vi "Periodic Tasks.vi"(8 "error in":errorcluster) -> ()   [LabVIEW 2015]
doc: "This VI runs in parallel to other tasks. It can contain as many user-defined periodic loops as you need. These can carry out PID or other sorts of timed response."
uses:
  Common Code/Goal Vision Packet.ctl
  Common Code/Change Detect Int.vi
  Common Code/Utilities/TimeManager.vi
  Common Code/Change Detect Boolean.vi
  Robot Global Data.vi
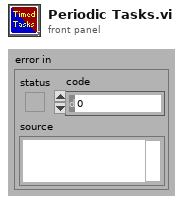
[diagram p1: front panel]
types:
  T1 = typedef "WPI_MotorControlDeviceRef.ctl" = cluster{"DeviceStatus":errorcluster, "Type":T2, "PWM":cluster{"PWM Channel":T3, "DeadBand":T4}, "CAN":cluster{"Device Number":u8, "Control Mode":T5, "Semaphore":T6, "Max Vout":dbl, "TalonSRX Control Mode":T7}, "Invert":bool}
  T2 = typedef "WPI_MotorControlType.ctl" = enum16{"PWM", "CAN", "CANTalonSRX"}
  T3 = typedef "FPGA_DIOPWMChannel.ctl" = enum8{"PWM 0", "PWM 1", "PWM 2", "PWM 3", "PWM 4", "PWM 5", "PWM 6", "PWM 7", "PWM 8", "PWM 9", "PWM MXP 0", "PWM MXP 1", "PWM MXP 2", "PWM MXP 3", "PWM MXP 4", "PWM MXP 5", "PWM MXP 6", "PWM MXP 7", "PWM MXP 8", "PWM MXP 9", "Invalid"}
  T4 = typedef "WPI_PWMDeadband.ctl" = cluster{"Name":string, "maxPositivePwm":i32, "minPositivePwm":i32, "centerPwm":i32, "maxNegativePwm":i32, "minNegativePwm":i32, "angularRange":u16}
  T5 = typedef "WPI_CANJaguar_ControlMode.ctl" = enum8{"Percent VBus", "Current", "Speed", "Position", "Voltage"}
  T6 = typedef "Semaphore RefNum" = refnum<k1>
  T7 = typedef "WPI_CANTalonSRX_APIControlMode.ctl" = enum8{"Percent VBus", "Speed", "Position", "Slave", "Unchanged / Invalid", "Voltage Compensation", "Current", "Motion Profile"}
  T8 = typedef "WPI_DriverStationRobotMode2.ctl" = enum16{"Autonomous Disabled", "Autonomous Enabled", "Teleop Disabled", "Teleop Enabled", "Disconnected", "Finish", "Test Disabled", "Test Enabled", "Emergency Stopped"}
  T9 = typedef "Shooter State Cluster.ctl" = cluster{"State":T10, "Left RPM":dbl, "Right RPM":dbl, "Shooter Ready?":bool, "Ball Loaded?":bool, "Current Angle":dbl, "Angle Motor Output":dbl, "Trigger Output":dbl, "Angle Ready?":bool, "RPM Ready?":bool, "Vision Ready?":bool, "Ball Loaded?":bool, "Mode":T11, "Shot Type":T12, "Pot Height":dbl, "Current Tripped Forward?":bool, "Current Tripped Backward?":bool, "Right Servo":i32, "Left Servo":i32, "IR Override":bool, "Intake Danger?":bool, "Intake Angle Ready?":bool}
  T10 = typedef "Shooter State.ctl" = enum16{"Idle", "Settle Ball", "Warmup", "Shooter Ready", "Shoot"}
  T11 = typedef "Shoot Modes Enum.ctl" = enum16{"Manual", "Safe", "Auto"}
  T12 = typedef "Shot Type.ctl" = enum16{"Batter Shot", "Corner Shot", "Cleat Shot", "Vision Shot", "Deep Middle Shot"}
  T13 = typedef "Goal Vision Packet.ctl" = cluster{"Distance":dbl, "Center X":dbl, "Center Y":dbl, "Found Target?":bool, "Robot Center":dbl, "Angle":dbl}
  T14 = typedef "Dashboard Control Data.ctl" = cluster{"Shooter Presets":T15, "Encoder Control":T17, "Steer PID output":cluster{"output high":dbl, "output low":dbl}, " Steer PID gains":cluster{"proportional gain (Kc)":dbl, "integral time (Ti, min)":dbl, "derivative time (Td, min)":dbl}, "Drivetrain Settings":T18, "Vision Packet":T13, "Dashboard Drivetrain Command":T19, "Info/Command Cluster":T21, "Ball Vision Packet":T22, "Intake Presets":T24, "Intake Encoder Control":T26, "Climb Presets":T27, "Goal Output Range":cluster{"output high":dbl, "output low":dbl}, "Enabled Systems":T28, "Auton Presets":T29, "Pressure M":dbl, "Pressure B":dbl, "Vision Timeout":dbl, "Auto-Shift":T30}
  T15 = typedef "Shooter Presets.ctl" = cluster{"Batter Shot":T16, "Deep Middle":T16, "Manual Shot":T16, "Left Ticks Per Rotation":dbl, "Right Ticks Per Rotation":dbl, "Low Bar Shot":T16, "Shooter RPM Tolerance":dbl, "Trigger Power":dbl, "Fire from Load Delay":i32, "Max Angle":dbl, "Min Angle":dbl, "Angle PID gains":cluster{"P":dbl, "I":dbl, "D":dbl}, "Angle Output":cluster{"output high":dbl, "output low":dbl}, "Shooter Angle Tolerance":dbl, "Vision Shoot x^2":dbl, "Vision Shoot x":dbl, "Feed Forward Max Accel":dbl, "Feed Forward Kv":dbl, "Backwards Trigger":dbl, "Shot Finish Delay (ms)":dbl, "Angle Max Current":dbl, "Angle Current Trip Time":dbl, "Intake Angle":dbl, "Vision Shoot c":dbl, "Reset?":bool, "Button Release Delay":dbl, "Angle Pot x":dbl, "Angle Pot c":dbl, "Ignore Angle?":bool, "Max RPM":dbl, "Safty Frist Angle":dbl, "Intake Danger Height":dbl, "Angle Pot B":i32, "Angle Pot M":dbl, "FF Finish RPM":dbl, "RPM PID Right":cluster{"P":dbl, "I":dbl, "D":dbl, "FF":dbl}, "RPM PID Left":cluster{"P":dbl, "I":dbl, "D":dbl, "FF":dbl}, "Backwards RPM":dbl, "Vision RPM":dbl, "Run Wheels Backward Delay":u32, "Cleat Shot":T16, "Vision Far RPM":dbl, "Vision Far Distance":dbl, "Vision Far Angle":dbl}
  T16 = typedef "Shot Presets.ctl" = cluster{"L":dbl, "R":dbl, "A":dbl}
  T17 = typedef "Encoder Control.ctl" = cluster{"Right Tick Constant":dbl, "Left Tick Constant":dbl, "Reset?":bool, "Y Dist":cluster{"PID gains":cluster{"proportional gain (Kc)":dbl, "integral time (Ti, min)":dbl, "derivative time (Td, min)":dbl}}, "Y Stop Thresh":dbl, "Y Stop Speed":dbl}
  T18 = typedef "Drivetrain Settings.ctl" = cluster{"Gyro Tolerance":dbl, "Throttle Ramp (ms)":dbl, "Kv":dbl, "Ka":dbl, "Feed Forward P":dbl, "Feed Forward D":dbl, "Goal Vision PID gains":cluster{"proportional gain (Kc)":dbl, "integral time (Ti, min)":dbl, "derivative time (Td, min)":dbl}, "Goal Detection Window":dbl, "Creep Rate":dbl, "Vision Throttle Threshold":dbl, "Min Turn Output":dbl, "Left Batter Angle":dbl, "Right Batter Angle":dbl}
  T19 = typedef "Dashboard Drivetrain Command.ctl" = cluster{"Drivetrain Vision":T20}
  T20 = typedef "Drivetrain Vision.ctl" = cluster{"Goal Window":dbl, "Ball Window":dbl}
  T21 = typedef "Ball Tracking Command Cluster.ctl" = cluster{"Distance to Ball":dbl, "Desired Angle":dbl, "Command":enum16{"Turn to Ball", "Turn to Angle", "Get Distance"}, "Pixels from Center":dbl}
  T22 = typedef "Ball Vision Packet.ctl" = cluster{"Ball Detected?":bool, "Distance to Ball":dbl, "Desired Angle":dbl, "Pixels from Center":dbl, "Tracking mode":T23}
  T23 = typedef "Tracking Mode.ctl" = enum16{"Turn to Ball", "Turn to Angle"}
  T24 = typedef "Intake Presets.ctl" = cluster{"Intake Speed":dbl, "Outake Speed":dbl, "Low Height":dbl, "Half Height":dbl, "High Idle Height":dbl, "Angle Speed":dbl, "Angle Tolerance":dbl, "Encoder Scale":dbl, "Load Height":dbl, "Output Range":T25, "Rotation Power Max/Min":dbl, "MaxCurrent":dbl, "Intake Trip Time":dbl, "Idle Height":dbl, "Max Height":dbl, "Reset Encoders?":bool, "PID gains":cluster{"proportional gain (Kc)":dbl, "integral time (Ti, min)":dbl, "derivative time (Td, min)":dbl}, "Intake Stop Delay":u32, "Settle Time":dbl, "Settle Wait Time":dbl, "Pull Up Delay":dbl}
  T25 = typedef "Drivetrain Output Range.ctl" = cluster{"output high":dbl, "output low":dbl}
  T26 = typedef "IntakeEcoderControl.ctl" = cluster{"Arm Tick Constant":dbl, "Reset?":bool, "Y Dist":cluster{"PID gains":cluster{"proportional gain (Kc)":dbl, "integral time (Ti, min)":dbl, "derivative time (Td, min)":dbl}}, "Y Stop Thresh":dbl, "Y Stop Speed":dbl}
  T27 = typedef "Climb Presets.ctl" = cluster{"Pull Power":dbl, "Extend Power":dbl}
  T28 = typedef "Enabled Systems.ctl" = cluster{"Shoot":bool, "Intake":bool, "DT":bool, "Gyro":bool, "100ms":bool, "US":bool}
  T29 = typedef "Autonomous Presets.ctl" = cluster{"Pitch Limit":dbl, "Roll Limit":dbl, "Start Position":dbl, "Cross Position":dbl}
  T30 = typedef "Auto Shift Cluster.ctl" = cluster{"Delay":dbl, "Speed Thresh":dbl, "Upshift Accel":dbl, "Upshift Throttle":dbl, "Upshift Throttle Accel":dbl, "Downshift Throttle":dbl, "Downshift Throttle Accel":dbl}
  T31 = typedef "WPI_CameraDevRef.ctl" = cluster{"Camera Address":string, "CameraStatus":errorcluster}
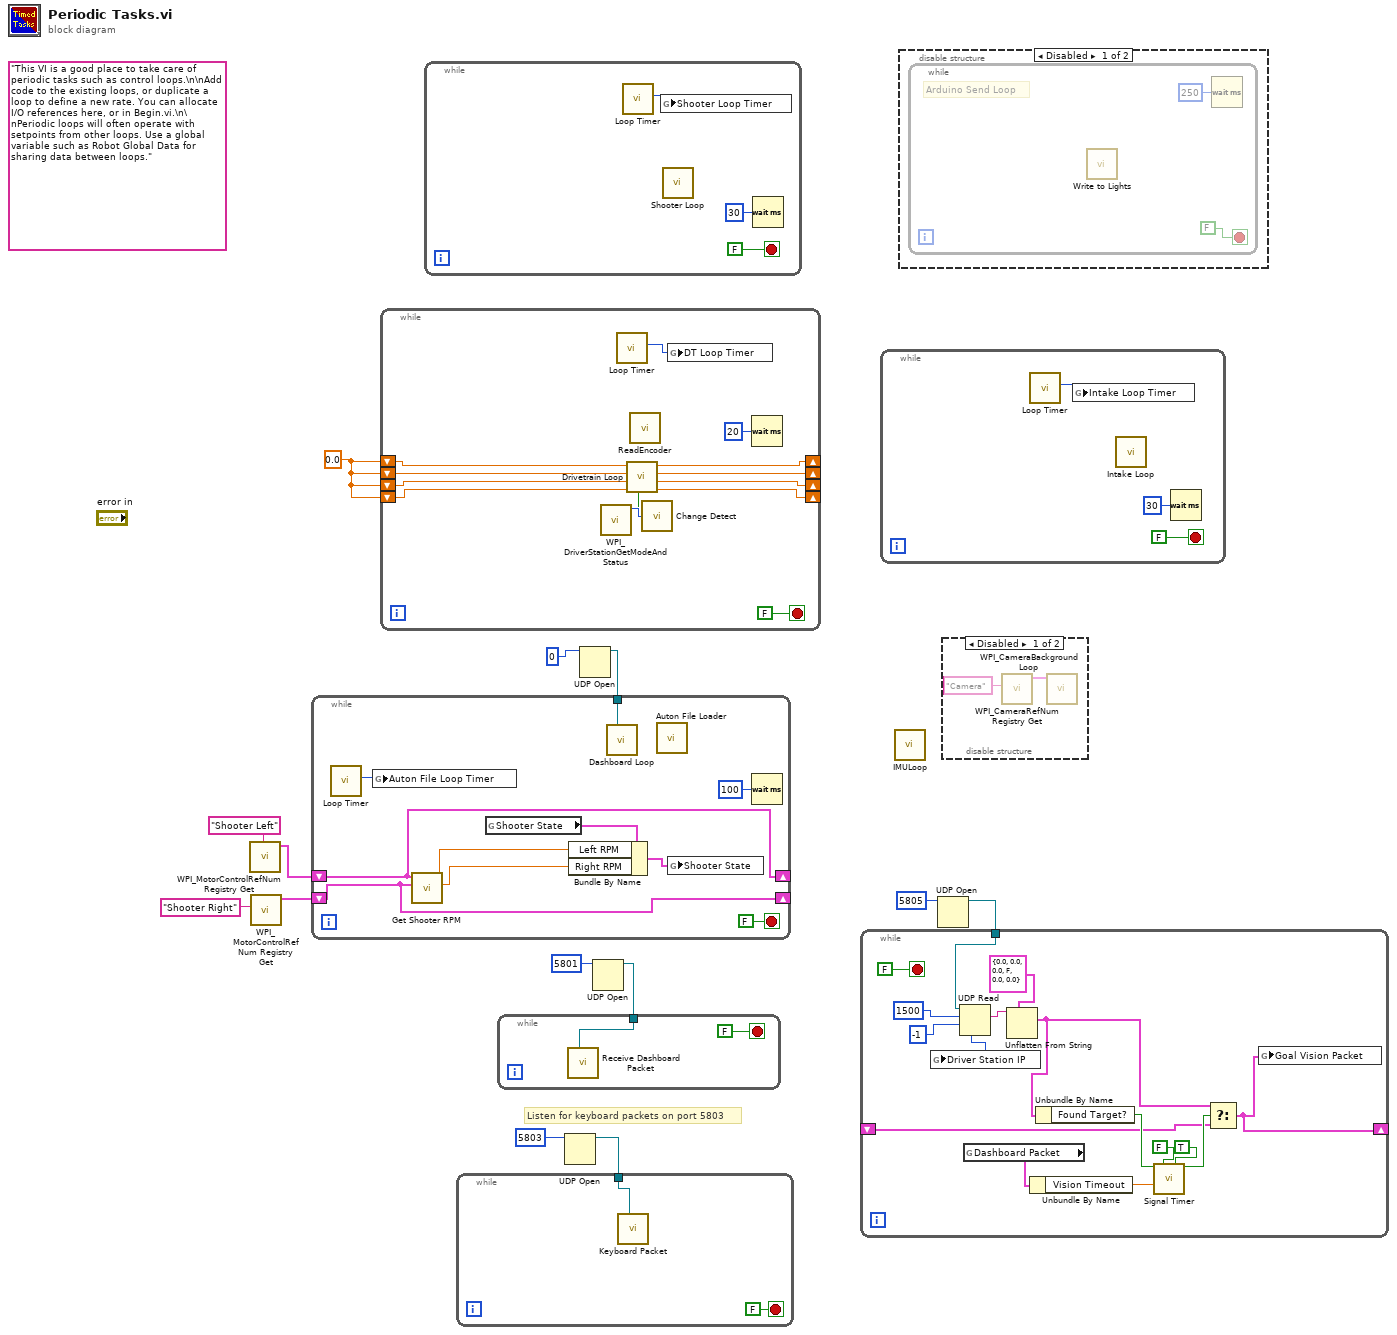
[diagram p0: block diagram]
diagram:
  w7 = 0.0 ("Timer 1 out")
  (unwired) "This VI is a good place to take care of periodic tasks such as control loops.\n\nAdd code to the existing loops, or duplicate a loop to define a new rate. You can allocate I/O references here, or in Begin.vi.\n\nPeriodic loops will often operate with setpoints from other loops. Use a global variable such as Robot Global Data for sharing data between loops."
  # "Listen for keyboard packets on port 5803"
  n1 = call <vilib>:"WPI_MotorControlRefNum Registry Get.vi"("refnum name"="Shooter Left") -> ("MotorControlDevRef"=w3:T1)  [unwired: 9 in, 1 out]
  n2 = call <vilib>:"WPI_MotorControlRefNum Registry Get.vi"("refnum name"="Shooter Right") -> ("MotorControlDevRef"=w4:T1)  [unwired: 9 in, 1 out]
  n3 = while {
    shift-right: [w19] -> _
    shift-left: w7 -> [w20]
    shift-right: [w23] -> _
    shift-left: w7 -> [w24]
    shift-right: [w18] -> _
    shift-left: w7 -> [w22]
    shift-right: [w17] -> _
    shift-left: w7 -> [w21]
    stop <- FALSE stop-if-true
    n4 = call <vilib>:"WPI_DriverStationGetModeAndStatus.vi"() -> ("Robot Mode"=w15:T8)  [unwired: 10 in, 1 out]
    n5 = call "Loop Timer.vi"() -> ("dt"=w16:u32)  [unwired: 11 in]
    n6 = call "ReadEncoder.vi"() -> ()  [unwired: 11 in, 1 out]
    n7 = call-poly "Change Detect.vi"("In"=w15) -> ("Changed?"=w14:bool)
    n8 = call "Drivetrain Loop.vi"("Reset the clock"=w14, "In 4"=w21, "In 3"=w22, "In 2"=w24, "In 1"=w20) -> ("Out 4"=w17:dbl, "Out 3"=w18:dbl, "Out 2"=w23:dbl, "Out 1"=w19:dbl)  [unwired: 3 in]
    n9 = global write "Robot Global Data.vi" "DT Loop Timer"(w16) -> ()
    n10 = Wait (ms)(milliseconds to wait=u32 20) -> ()  [unwired: 1 out]
  }
  n11 = while {
    stop <- FALSE stop-if-true
    n12 = call "Loop Timer.vi"() -> ("dt"=w27:u32)  [unwired: 11 in]
    n13 = global write "Robot Global Data.vi" "Shooter Loop Timer"(w27) -> ()
    n14 = call "Shooter Loop.vi"() -> ()  [unwired: 12 in]
    n15 = Wait (ms)(milliseconds to wait=u32 30) -> ()  [unwired: 1 out]
  }
  n16 = UDP Open(11:u16 5803 ("port")) -> (port=w8:refnum<k16>)  [unwired: 4 in, 2 out]
  n17 = while {
    tunnel: w8 -> [w30]
    stop <- FALSE stop-if-true
    n18 = call "Keyboard Packet.vi"("connection ID"=w30) -> ()  [unwired: 11 in]
  }
  n19 = UDP Open(11:0) -> (port=w11:refnum<k16>)  [unwired: 4 in, 2 out]
  n20 = while {
    tunnel: w11 -> [w39]
    shift-right: [w32] -> _
    shift-left: w3 -> [w32]
    shift-right: [w33] -> _
    shift-left: w4 -> [w33]
    stop <- FALSE stop-if-true
    n21 = call "Loop Timer.vi"() -> ("dt"=w38:u32)  [unwired: 11 in]
    n22 = global write "Robot Global Data.vi" "Auton File Loop Timer"(w38) -> ()
    n23 = call "Get Shooter RPM.vi"("Shooter Right"=w33, "Shooter Left"=w32) -> ("Right RPM"=w35:dbl, "Left RPM"=w36:dbl)  [unwired: 5 in, 3 out]
    n24 = global read "Robot Global Data.vi" "Shooter State"() -> (w37:T9)
    n25 = Bundle By Name(cluster=w37, "Left RPM"=w36, "Right RPM"=w35) -> (w34:T9)
    n26 = call "Dashboard Loop.VI"("connection ID"=w39) -> ()  [unwired: 11 in]
    n27 = call "Auton File Loader.vi"() -> ()  [unwired: 12 in]
    n28 = global write "Robot Global Data.vi" "Shooter State"(w34) -> ()
    n29 = Wait (ms)(milliseconds to wait=u32 100) -> ()  [unwired: 1 out]
  }
  n30 = UDP Open(11:u16 5801 ("port")) -> (port=w13:refnum<k16>)  [unwired: 4 in, 2 out]
  n31 = while {
    tunnel: w13 -> [w42]
    stop <- FALSE stop-if-true
    n32 = call "Receive Dashboard Packet.vi"("connection ID"=w42) -> ()  [unwired: 11 in]
  }
  n33 = while {
    stop <- FALSE stop-if-true
    n34 = call "Loop Timer.vi"() -> ("dt"=w44:u32)  [unwired: 11 in]
    n35 = global write "Robot Global Data.vi" "Intake Loop Timer"(w44) -> ()
    n36 = call "Intake Loop.vi"() -> ()  [unwired: 12 in]
    n37 = Wait (ms)(milliseconds to wait=u32 30) -> ()  [unwired: 1 out]
  }
  n38 = call "IMULoop.vi"() -> ()  [unwired: 12 in]
  n39 = disable-structure shown="Disabled" {
    frame Disabled {
      n40 = while {
        stop <- FALSE stop-if-true
        # "Arduino Send Loop"
        n41 = call "Write to Lights.vi"() -> ()  [unwired: 12 in]
        n42 = Wait (ms)(milliseconds to wait=u32 250) -> ()  [unwired: 1 out]
      }
    }
    frame Enabled {
    }
  }
  n43 = UDP Open(11:u16 5805 ("port")) -> (port=w2:refnum<k16>)  [unwired: 4 in, 2 out]
  n44 = while {
    tunnel: w2 -> [w64]
    shift-right: [w57] -> _
    shift-left: _ -> [w50]
    stop <- FALSE stop-if-true
    n45 = UDP Read(connection ID=w64, max size (548)=1500, timeout ms (25000)=-1) -> (data out=w63:string, 6:w62:u32)  [unwired: 1 in, 3 out]
    n46 = global write "Robot Global Data.vi" "Driver Station IP"(w62) -> ()
    n47 = global read "Robot Global Data.vi" "Dashboard Packet"() -> (w53:T14)
    n48 = Unflatten From String(type=T13 {"Distance"=0.0, "Center X"=0.0, "Center Y"=0.0, "Found Target?"=FALSE, "Robot Center"=0.0, "Angle"=0.0} ("Goal Vision Packet"), binary string=w63) -> (value=w59:T13)  [unwired: 3 in, 2 out]
    n49 = Unbundle By Name(w53) -> ("Vision Timeout"=w54:dbl)
    n50 = Unbundle By Name(w59) -> ("Found Target?"=w55:bool)
    n51 = call "Signal Timer.vi"("Input"=w55, "Edge"=FALSE, "Interval"=w54, "Pull"=TRUE) -> ("Filtered Output"=w56:bool)  [unwired: 11 in]
    n52 = Select(t=w59, s=w56, f=w50) -> (s? t:f=w57:T13)
    n53 = global write "Robot Global Data.vi" "Goal Vision Packet"(w57) -> ()
  }
  n54 = disable-structure shown="Disabled" {
    frame Disabled {
      n55 = call <vilib>:"WPI_CameraRefNum Registry Get.vi"("refnum name"="Camera") -> ("CameraDevRef"=w65:T31)  [unwired: 9 in, 1 out]
      n56 = call <vilib>:"WPI_CameraBackground Loop.vi"("CameraDevRef"=w65) -> ()  [unwired: 11 in]
    }
    frame Enabled {
    }
  }
